vi "LibXML_EliminatePredefinedEntities.vi"(8 "error in":errorcluster, 9 "Replacements":string[](array[string])=["&amp;", "&gt;", "&lt;"], 10 "Chars to Replace":string[](array[string])=["&", ">", "<"], 11 "XML text":string) -> (0 "error out":errorcluster, 3 "XML (escaped)":string)   [LabVIEW 2019, in "Tools.lvlib"]
doc: "Escapes &, >, and < for XML standards."
uses:
  Tools.lvlib
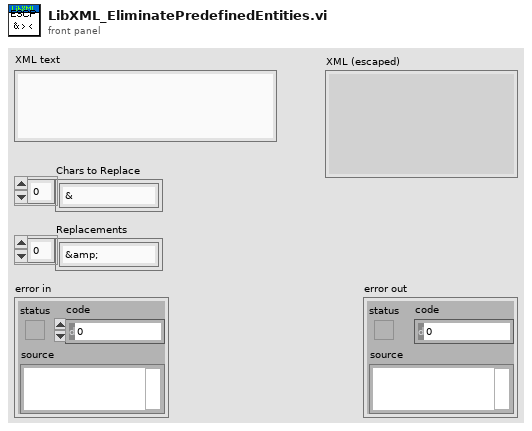
[diagram p1: front panel]
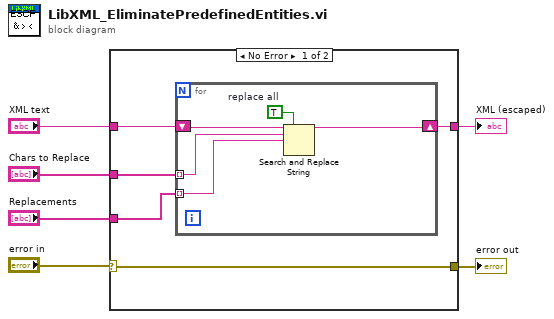
[diagram p0: block diagram]
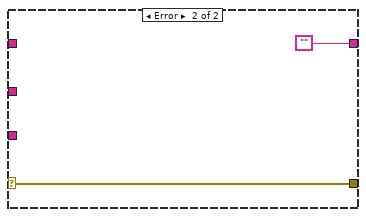
[diagram p2: hidden frame]
diagram:
  n1 = case shown="No Error" "error in" {
    selector: "error in" -> [w7 w17]
    tunnel: "XML text" -> [w11 _]
    tunnel: "Chars to Replace" -> [w10 _]
    tunnel: "Replacements" -> [w9 _]
    tunnel: [w8 "" ("XML text")] -> w3
    tunnel: [w7 w17] -> w1
    frame No Error {
      n2 = for {
        shift-right: [w12] -> w8
        shift-left: w11 -> [w16]
        tunnel: w10 -> [w15] mode=indexing
        tunnel: w9 -> [w14] mode=indexing
        w13 = TRUE  # replace all
        n3 = Search and Replace String(replace all?=w13, input string=w16, search string=w15, replace string=w14) -> (result string=w12:string)  [unwired: 4 in, 3 out]
      }
    }
    frame Error {
    }
  }
  "XML (escaped)" <- w3
  "error out" <- w1
